vi "Get All Events in Module.vi"(7 "include all events (F)":bool, 8 "error in (no error)":errorcluster, 11 "Module Info":T1) -> (0 "error out":errorcluster, 3 "Event Info":T2(array[cluster]))   [LabVIEW 2020, in "DQMH_API.lvclass"]
uses:
  <resource>/Framework/Providers/Open_GDS/UML/DQMH_API_class/DQMH_API.lvclass
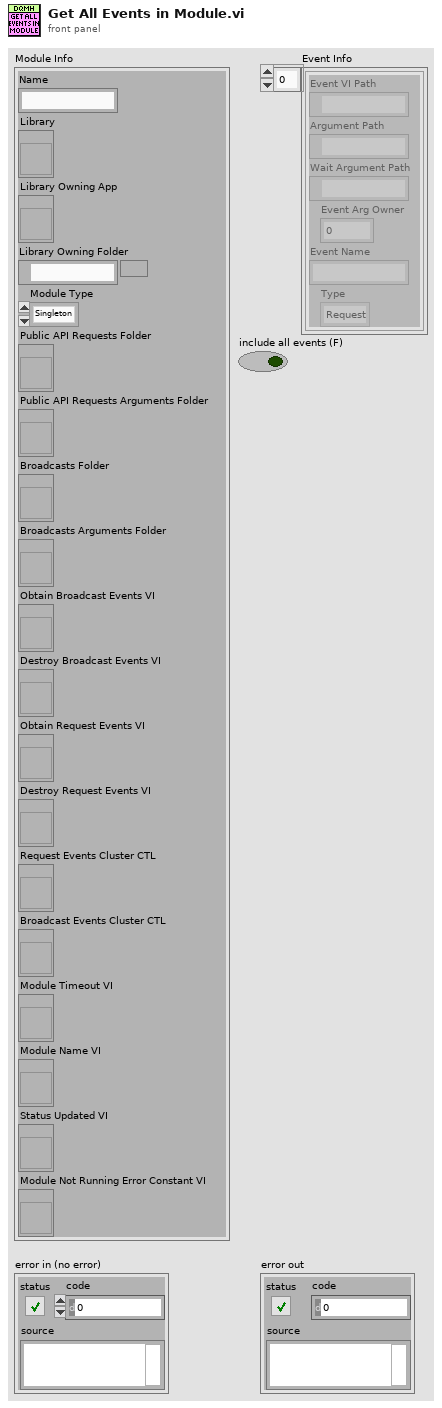
[diagram p1: front panel]
types:
  T1 = cluster{"Name":string, "Library":refnum<vi>, "Library Owning App":refnum<vi>, "Library Owning Folder":path, "Module Type":enum16{"Singleton", "Cloneable"}, "Public API Requests Folder":refnum<vi>, "Public API Requests Arguments Folder":refnum<vi>, "Broadcasts Folder":refnum<vi>, "Broadcasts Arguments Folder":refnum<vi>, "Obtain Broadcast Events VI":refnum<vi>, "Destroy Broadcast Events VI":refnum<vi>, "Obtain Request Events VI":refnum<vi>, "Destroy Request Events VI":refnum<vi>, "Request Events Cluster CTL":refnum<vi>, "Broadcast Events Cluster CTL":refnum<vi>, "Module Timeout VI":refnum<vi>, "Module Name VI":refnum<vi>, "Status Updated VI":refnum<vi>, "Module Not Running Error Constant VI":refnum<vi>}
  T2 = cluster{"Event VI Path":path, "Argument Path":path, "Wait Argument Path":path, "Event Arg Owner":i32, "Event Name":string, "Type":enum16{"Request", "Broadcast", "Both"}}[]
  T3 = typedef "DQMH_API.lvclass/ObjectAttributes.ctl" = cluster{"Get Module Type Info":refnum<vi>, "Script New Module":refnum<vi>, "Script New Event":refnum<vi>, "Query Library for Module Info":refnum<vi>, "Parse Project for DQMH Modules":refnum<vi>, "Get All Events in Module":refnum<vi>}
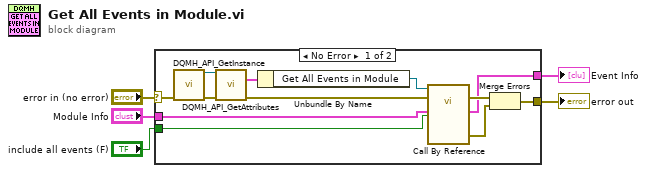
[diagram p0: block diagram]
diagram:
  n1 = case shown="No Error" "error in (no error)" {
    selector: "error in (no error)" -> [w15 w18]
    tunnel: [w7 w18] -> w4
    tunnel: "include all events (F)" -> [w10 _]
    tunnel: "Module Info" -> [w9 _]
    tunnel: [w8 _] -> w1
    frame No Error {
      n2 = call <resource>:"DQMH_API_GetInstance.vi"("error in (no error)"=w15) -> ("reference out"=w16:refnum<class "DQMH_API.lvclass">, "error out"=w14:errorcluster)  [unwired: 10 in, 3 out]
      n3 = call <resource>:"DQMH_API_GetAttributes.vi"("reference in"=w16, "error in (no error)"=w14) -> ("Data"=w17:T3, "error out"=w12:errorcluster)  [unwired: 10 in, 2 out]
      n4 = Unbundle By Name(w17) -> ("Get All Events in Module"=w13:refnum<vi>)
      n5 = call-by-ref "?"(reference=w13, error in=w12, "include all events (F)"=w10, "Module Info"=w9) -> (error out=w11:errorcluster, 0:"error out"=w6:errorcluster, "Event Info"=w8:T2)  [unwired: 8 in, 1 out]
      n6 = Merge Errors(w11, w6) -> (w7:errorcluster)
    }
    frame Error {
    }
  }
  "error out" <- w4
  "Event Info" <- w1
